vi "DBInsertToTable-Log.vi"(8 "error in (no error)":errorcluster, 9 "message value":variant, 11 "ProcessState in":T1) -> (0 "error out":errorcluster, 3 "ProcessState out":T1)   [LabVIEW 2015, in "CopyUtility.lvlib"]
uses:
  CopyUtility.lvlib
  controls/ProcessState.ctl
  <vilib>/drjdpowell/SQLite Library/SQL Connection/Connection.lvclass
  <vilib>/drjdpowell/SQLite Library/SQL Statement/SQL Statement.lvclass/SQL Statement.ctl
  <vilib>/drjdpowell/SQLite Library/SQL Statement/Bind Timestamp (Text).vi
  <vilib>/drjdpowell/SQLite Library/SQL Statement/Bind Text.vi
  <vilib>/drjdpowell/SQLite Library/SQL Statement/Bind Integer.vi
  <vilib>/drjdpowell/SQLite Library/SQL Statement/Error Message.vi
  <vilib>/drjdpowell/SQLite Library/SQL Statement/SQL Statement.lvclass
  DBToolkit/DBToolkit.lvlib
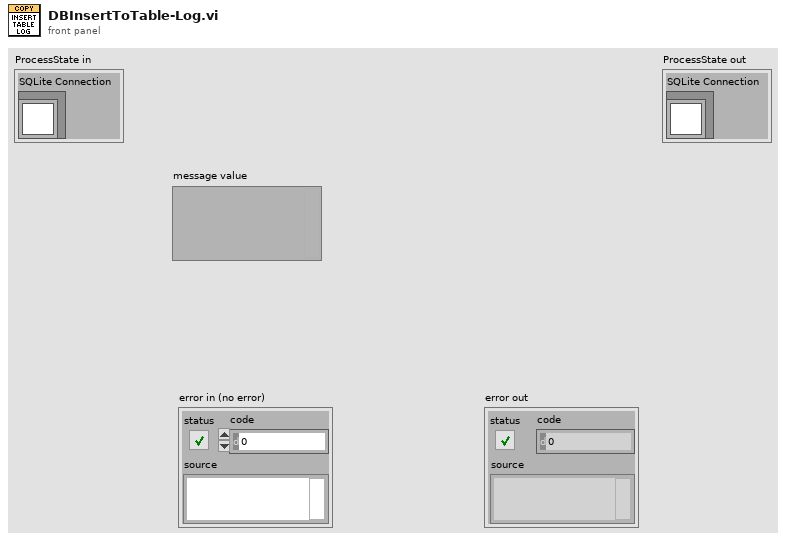
[diagram p1: front panel]
types:
  T1 = typedef "CopyUtility.lvlib/ProcessState.ctl" = cluster{"SQLite Connection":refnum<class "Connection.lvclass">}
  T2 = typedef "CopyUtility.lvlib/ErrorMessgae.ctl" = cluster{"Time":timestamp, "Source":string, "ErrorString":string, "Code":i32}
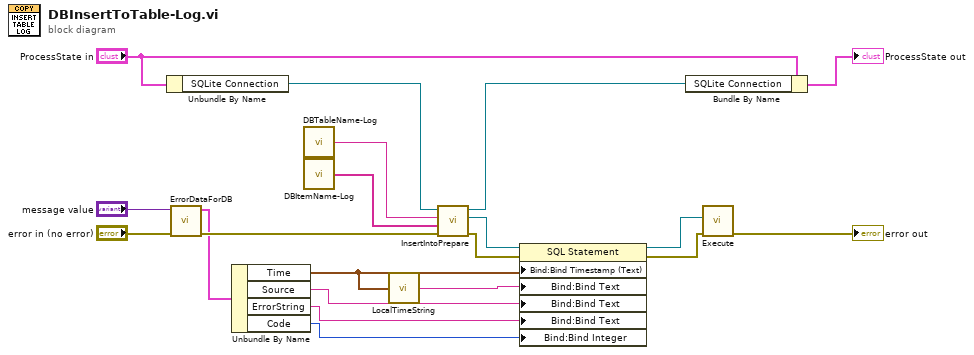
[diagram p0: block diagram]
diagram:
  n1 = Unbundle By Name("ProcessState in") -> ("SQLite Connection"=w18:refnum<class "Connection.lvclass">)
  n2 = call "ErrorDataForDB.vi"("error in (no error)"="error in (no error)", "process error message"="message value") -> ("error out"=w14:errorcluster, "ErrorMessage"=w13:T2)  [unwired: 8 in]
  n3 = Unbundle By Name(w13) -> ("Time"=w6:timestamp, "Source"=w10:string, "ErrorString"=w9:string, "Code"=w8:i32)
  n4 = call "DBTableName-Log.vi"() -> ("DB Table Name"=w5:string)  [unwired: 5 in]
  n5 = call "DBItemName-Log.vi"() -> ("Items"=w4:string[])  [unwired: 5 in]
  n6 = call "LocalTimeString.vi"("Time Stamp"=w6) -> ("Local Time String"=w7:string)  [unwired: 4 in]
  n7 = call "InsertIntoPrepare.vi"("error in (no error)"=w14, "Items"=w4, "Table Name"=w5, "SQLite Connection in"=w18) -> ("error out"=w20:errorcluster, "SQL Statement out"=w19:refnum<class "SQL Statement.lvclass">, "SQLite Connection out"=w17:refnum<class "Connection.lvclass">)  [unwired: 5 in]
  n8 = property class="SQL Statement"(reference=w19, error in=w20, "Bind:Bind Timestamp (Text)"=w6, "Bind:Bind Text"=w7, "Bind:Bind Text"=w10, "Bind:Bind Text"=w9, "Bind:Bind Integer"=w8) -> (reference out=w2:refnum<class "SQL Statement.lvclass">, error out=w1:errorcluster)
  n9 = Bundle By Name(cluster="ProcessState in", "SQLite Connection"=w17) -> (→"ProcessState out":T1)
  n10 = call "Execute.vi"("error in (no error)"=w1, "SQL Statement in"=w2) -> ("error out"=→"error out":errorcluster)  [unwired: 9 in]
